vi "去除野值.vi"(1 "输入数组":dbl[](array[numeric])=[-8888.0, -25.0, 24.0, 53.0, 56.0, 60.0, 1000.0]) -> (0 "去野数组":dbl[](array[numeric]))   [LabVIEW 2017]
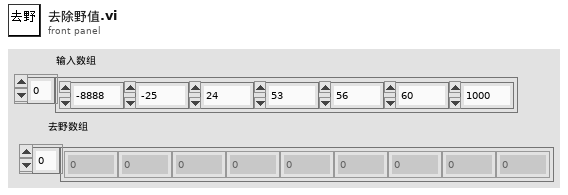
[diagram p1: front panel]
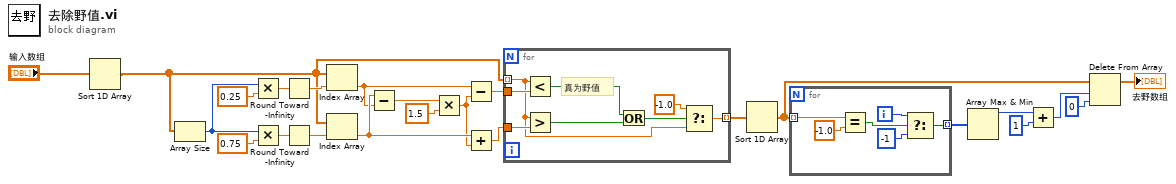
[diagram p0: block diagram]
diagram:
  n1 = Sort 1D Array(array="输入数组") -> (sorted array=w1:dbl[])
  n2 = Array Size(array=w1) -> (size(s)=w22:i32)
  n3 = Multiply(x=w22, y=0.25) -> (x*y=w20:dbl)
  n4 = Multiply(x=w22, y=0.75) -> (x*y=w21:dbl)
  n5 = Round Toward -Infinity(1:w20) -> (0:w18:dbl)
  n6 = Round Toward -Infinity(1:w21) -> (0:w19:dbl)
  n7 = Index Array(array=w1, index=w18) -> (element=w14:dbl)
  n8 = Index Array(array=w1, index=w19) -> (element=w15:dbl)
  n9 = Subtract(x=w15, y=w14) -> (x-y=w16:dbl)
  n10 = Multiply(x=w16, y=1.5) -> (x*y=w13:dbl)
  n11 = Subtract(x=w14, y=w13) -> (x-y=w11:dbl)
  n12 = Add(x=w15, y=w13) -> (x+y=w12:dbl)
  n13 = for {
    tunnel: w12 -> [w32]
    tunnel: w11 -> [w31]
    tunnel: w1 -> [w26] mode=indexing
    tunnel: [w25] -> w10 mode=indexing
    # "真为野值"
    n14 = Less?(x=w26, y=w31) -> (x < y?=w30:bool)
    n15 = Greater?(x=w26, y=w32) -> (0:w29:bool)
    n16 = Or(x=w30, y=w29) -> (x .or. y?=w28:bool)
    n17 = Select(t=-1.0, s=w28, f=w26) -> (s? t:f=w25:dbl)
  }
  n18 = Sort 1D Array(array=w10) -> (sorted array=w3:dbl[])
  n19 = for {
    tunnel: w3 -> [w38] mode=indexing
    tunnel: [w33] -> w9 mode=indexing
    i -> [w35]
    n20 = Equal?(x=w38, y=-1.0) -> (x = y?=w36:bool)
    n21 = Select(t=w35, s=w36, f=-1) -> (s? t:f=w33:i32)
  }
  n22 = Array Max & Min(array=w9) -> (max value=w8:i32)  [unwired: 3 out]
  n23 = Add(x=w8, y=1) -> (x+y=w6:i32)
  n24 = Delete From Array(array=w3, length=w6, index=0 ("索引")) -> (array with subset deleted=→"去野数组":dbl[])  [unwired: 1 out]
